vi "field emission sensor_v57.vi"() -> ()   [LabVIEW 2014]
uses:
  Keithley 24XX/Public/Data/Read (Single Point).vi
  Keithley 24XX/Keithley 24XX.lvlib
  <userlib>/Nanonis Prog Interface V5/Nanonis Prog Interface.lvlib
panel:
  out "amplitude":sgl(graph)
  in  "delay  coarse step":u32
  in  "Amplitude (V) (NaN=no change)":sgl=nan
  in  "Frequency (Hz) (NaN=no change)":sgl=nan format="%#_6p"
  in  "retract":dbl=2e-08 format="%#_6p"
  in  "amplitude max":sgl=1e-10 format="%#_6p"
  in  "Signal index (0-79)":i8=49
  out "amplitude":sgl=7.943678e-12 format="%#_6p"
  in  "dz":dbl=1e-09 format="%#_6p"
  in  "ramp delay":u16=10500
  out "ramp":bool
  out "millisecond timer value":u32=183946603
  in  "Clear plots":bool
  out "z":dbl(graph)=1.0959994182086754e-07
  in  "Ramp":bool=TRUE
  in  "steps":sgl=5e-09 format="%#_6p"
  in  "Ramp to":sgl=2.45e-07 format="%#_6p"
  in  "I":sgl=5e-05 format="%#_6p"
  in  "PID":bool
  in  "p":sgl=0.005 format="%#_6p"
  in  "setpoint":sgl=2.5000006e-07 format="%#_6p"
  in  "max Current":sgl=1e-06 format="%#_6p"
  in  "setpoint approach":sgl=3e-08 format="%#_6p"
  in  "auto approach":bool
  in  "Number of steps":u16=1
  in  "withdraw tip":bool
  in  "coarse step":bool
  in  "Direction":enum16{"X +", "X -", "Y +", "Y -", "Z +", "Z -"}(ring)=enum."Z +"
  in  "Machine name (local machine IP)":string="localhost"
  in  "Z position [m]":dbl=1.0959994182086754e-07 step=1.0 format="%_6p"
  out "current [A]":sgl=2.086008e-11 format="%#_6p"
  in  "time divider":dbl=60.0
  out "time elapsed":dbl=58.44645961125692
  in  "milliseconds to wait":u32=100
  in  "VISA resource name":refnum<visa-resource-name>="GPIB0::21::INSTR"
  in  "stop":bool
  in  "current multiplier":sgl=1.0
  out "Current":sgl(graph)=2.086008e-11
  # "STOP the VI during an Nanonis Auto Approach"
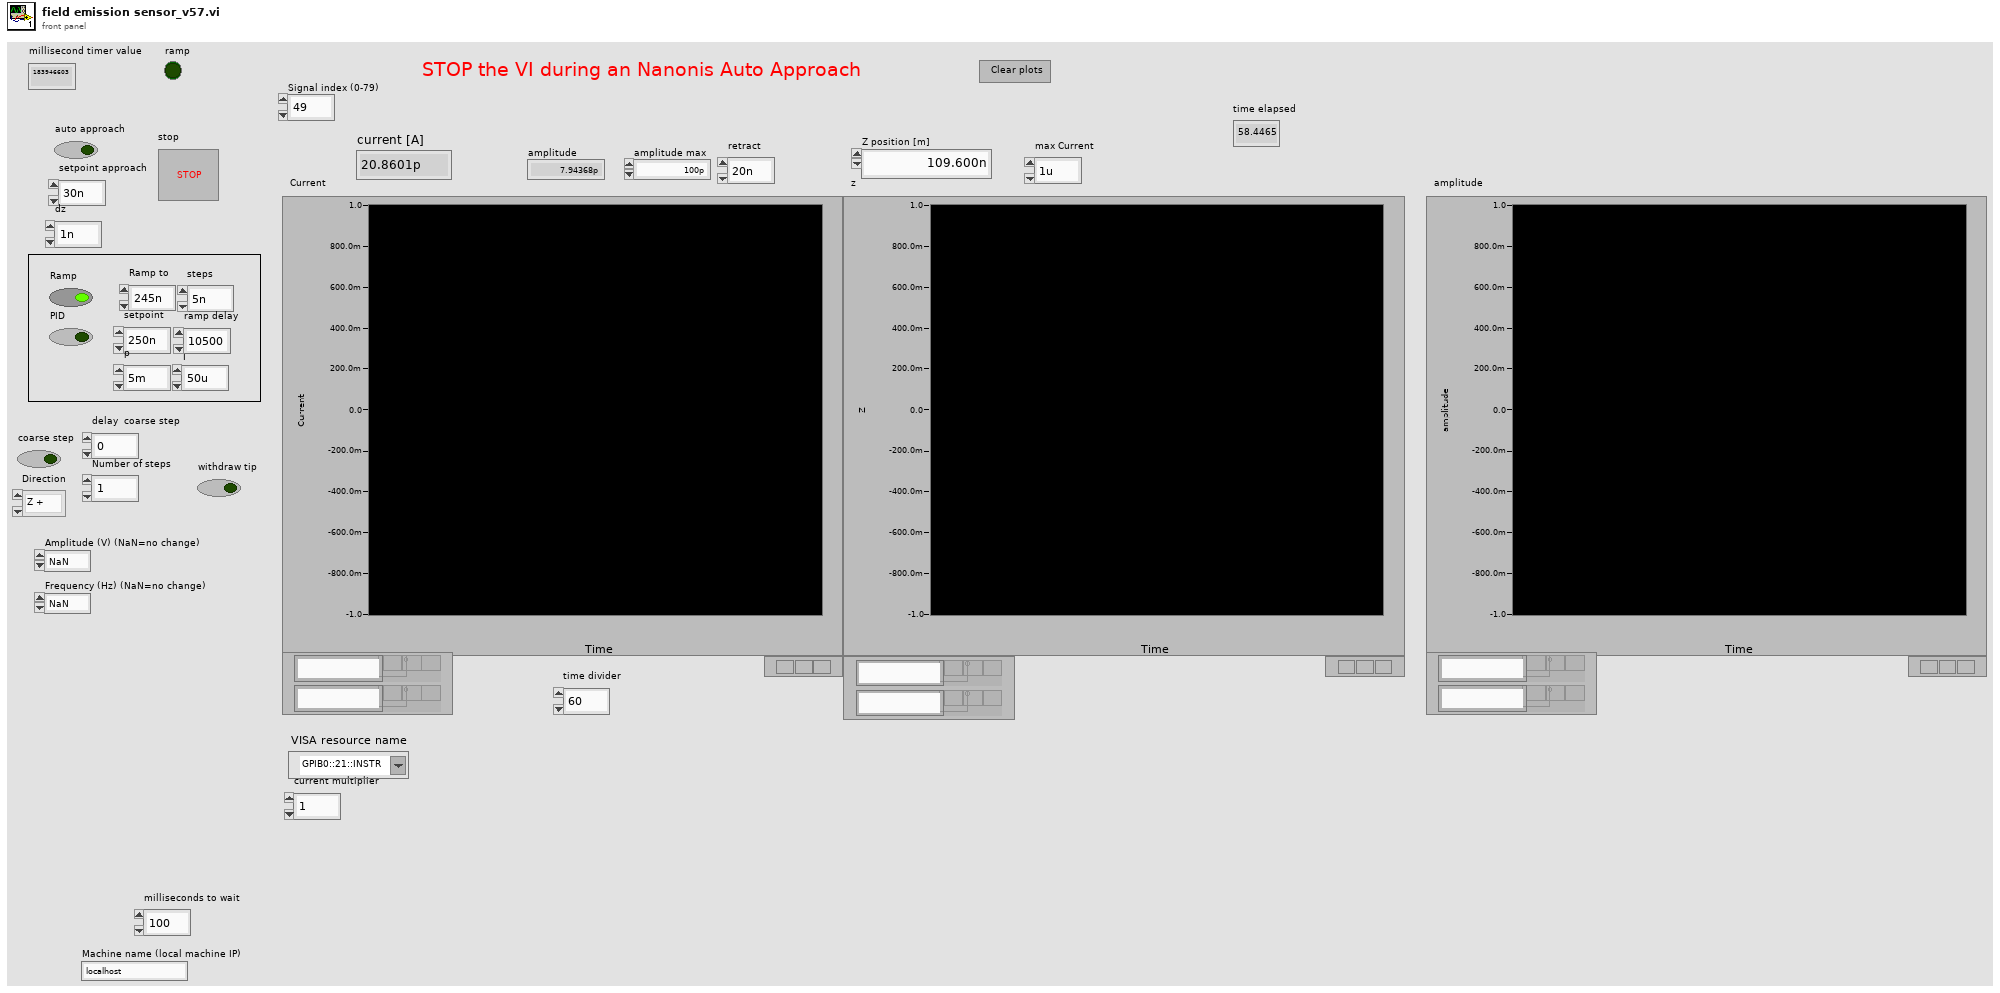
[diagram p1: front panel]
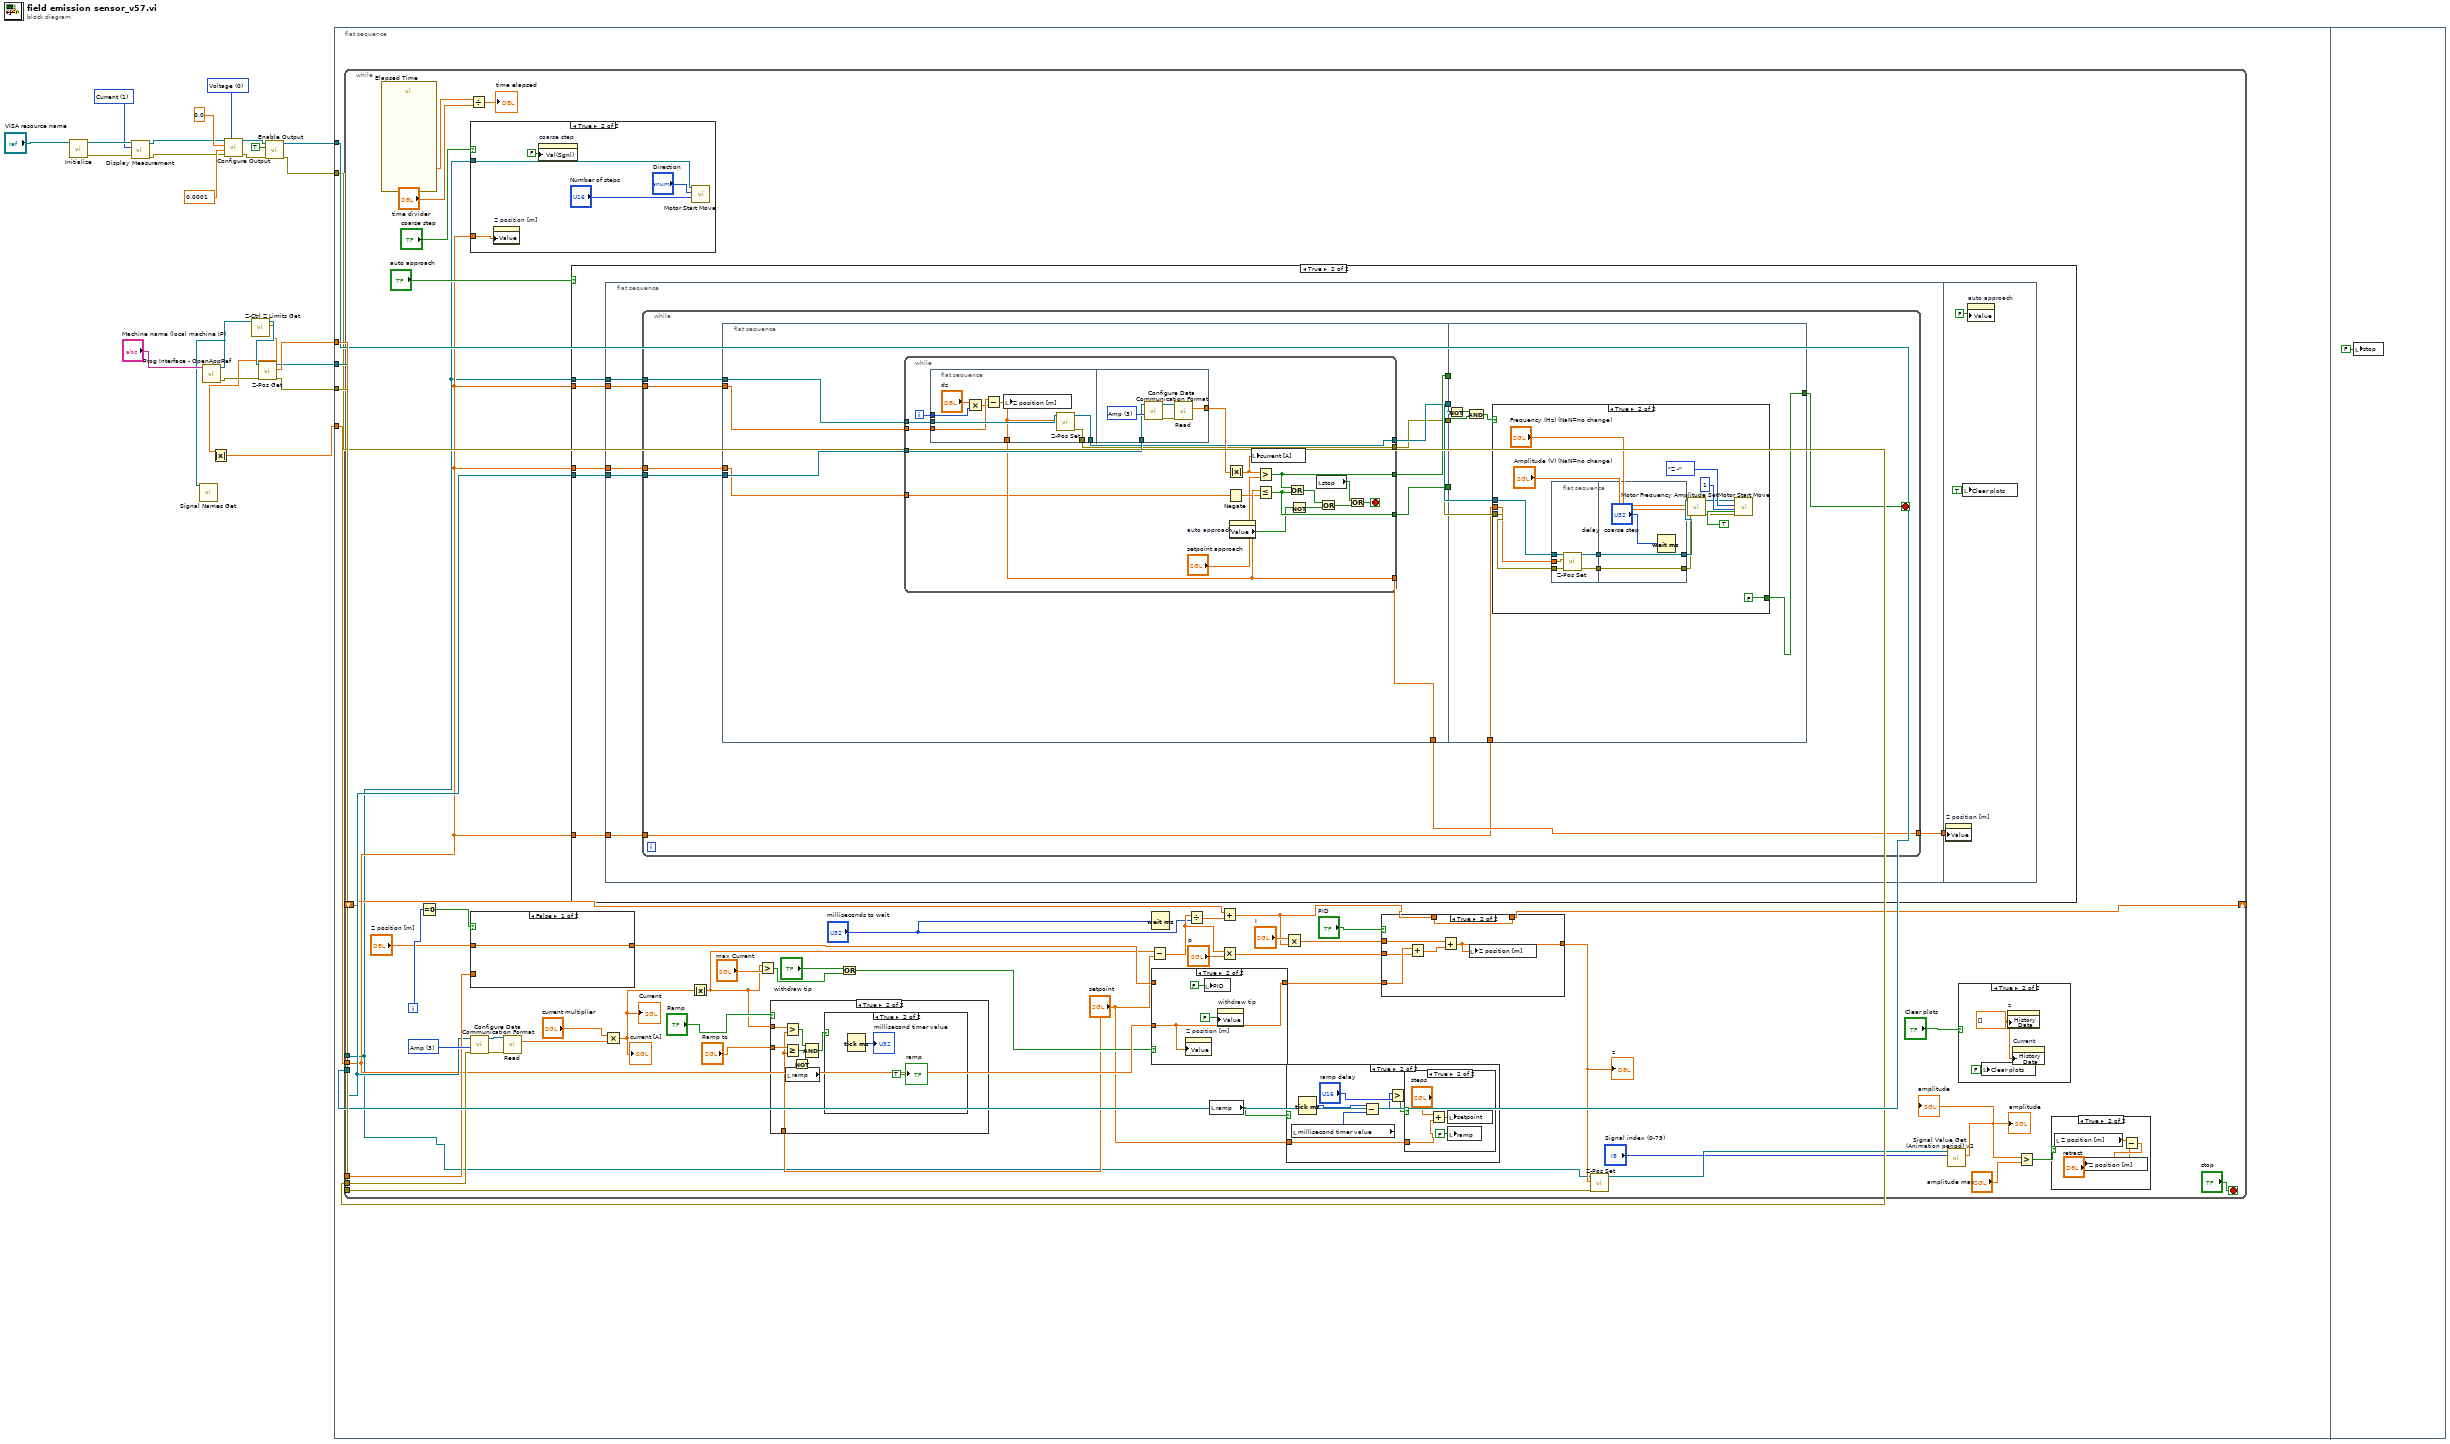
[diagram p0: block diagram]
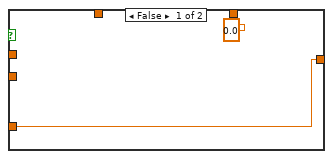
[diagram p8: hidden frame]
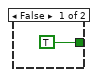
[diagram p10: hidden frame]
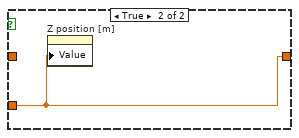
[diagram p13: hidden frame]
diagram:
  w5 = u16 1 items=["Voltage", "Current", "Resistance"] ("Displayed Measurement (0: Voltage)")
  w17 = u16 0 items=["Voltage", "Current"] ("Source Mode  (0: Voltage)")
  n1 = call "Initialize.vi"("VISA resource name"="VISA resource name") -> ("error out"=w7:errorcluster, "VISA resource name out"=w9:refnum<visa-resource-name>)  [unwired: 9 in]
  n2 = call "Display Measurement.vi"("error in (no error)"=w7, "Displayed Measurement (0: Voltage)"=w5, "VISA resource name"=w9) -> ("error out"=w6:errorcluster, "VISA resource name out"=w8:refnum<visa-resource-name>)  [unwired: 7 in]
  n3 = call <userlib>:"Prog Interface - OpenAppRef.vi"("Machine name (local machine IP)"="Machine name (local machine IP)") -> ("Error out"=w22:errorcluster, "Application reference"=w1:refnum<vi>)  [unwired: 5 in]
  n4 = call <userlib>:"Signal Names Get.vi"("Application ref in"=w1) -> ()  [unwired: 6 in, 3 out]
  n5 = call "Configure Output.vi"("Source Mode  (0: Voltage)"=w17, "error in (no error)"=w6, "Compliance  Level (0.1)"=0.0001, "Output Level (0)"=0.0, "VISA resource name"=w8) -> ("error out"=w13:errorcluster, "VISA resource name out"=w14:refnum<visa-resource-name>)  [unwired: 5 in]
  n6 = call <userlib>:"Z-Ctrl Z Limits Get.vi"("Application ref in"=w1) -> ("Z high limit"=w2:sgl, "Application ref out"=w3:refnum<vi>)  [unwired: 7 in, 2 out]
  n7 = Absolute Value(x=w2) -> (abs(x)=w4:sgl)
  n8 = call <userlib>:"Z-Pos Get.vi"("error in (no error)"=w22, "Application ref in"=w3) -> ("error out"=w21:errorcluster, "Z position (m)"=w20:sgl, "Application ref out"=w19:refnum<vi>)  [unwired: 7 in]
  n9 = call "Enable Output.vi"("error in (no error)"=w13, "Enable Output (T: Enable)"=TRUE, "VISA resource name"=w14) -> ("error out"=w10:errorcluster, "VISA resource name out"=w11:refnum<visa-resource-name>)  [unwired: 7 in]
  n10 = flat-sequence {
    tunnel: w21 -> [w29]
    tunnel: w20 -> [w28]
    tunnel: w19 -> [w27]
    tunnel: w11 -> [w26]
    tunnel: w10 -> [w25]
    tunnel: w4 -> [w24]
    frame #0 {
      n11 = while {
        tunnel: w27 -> [w33]
        tunnel: w29 -> [w71]
        tunnel: w28 -> [w70]
        tunnel: w26 -> [w62]
        tunnel: w25 -> [w61]
        tunnel: w24 -> [w59]
        shift-right: [w43] -> _
        shift-left: _ -> [w50]
        i -> [w69]
        stop <- "stop" stop-if-true
        w75 = u16 3 items=["All", "Volt and Amp", "Volt", "Amp"] ("Data Selection (0: All)")
        n12 = call "Elapsed Time"() -> ("Elapsed Time (s)"=w72:dbl)  [unwired: 12 in, 7 out]
        n13 = Equal To 0?(x=w69) -> (x = 0?=w68:bool)
        n14 = Divide(x=w72, y="time divider") -> (x/y=→"time elapsed":dbl)
        n15 = case shown="True" "coarse step" {
          tunnel: w33 -> [_ w221]
          tunnel: w59 -> [_ w217]
          frame False {
          }
          frame True {
            n16 = property on="Z position [m]" class="DigNum (strict)"("Value"=w217) -> ()  [unwired: 2 in, 2 out]
            n17 = property on="coarse step" class="Bool (strict)"("Val(Sgnl)"=FALSE ("Value (Signaling)")) -> ()  [unwired: 2 in, 2 out]
            n18 = call <userlib>:"Motor Start Move.vi"("Number of steps"="Number of steps", "Direction"="Direction", "Application ref in"=w221) -> ()  [unwired: 6 in, 2 out]
          }
        }
        n19 = case shown="False" w68 {
          tunnel: [w222 w223] -> w65
          tunnel: w70 -> [_ w223]
          tunnel: "Z position [m]" -> [w222 _]
          frame False {
          }
          frame True {
            n20 = property on="Z position [m]" class="DigNum (strict)"("Value"=w223) -> ()  [unwired: 2 in, 2 out]
          }
        }
        n21 = call "Configure Data Communication Format.vi"("error in (no error)"=w61, "Data Selection (0: All)"=w75, "VISA resource name"=w62) -> ("error out"=w76:errorcluster, "VISA resource name out"=w77:refnum<visa-resource-name>)  [unwired: 7 in]
        n22 = call-poly "Read.vi"("VISA resource name"=w77, "error in (no error)"=w76) -> ("Current"=w79:sgl)  [unwired: 7 in, 6 out]
        n23 = case shown="True" "auto approach" {
          tunnel: w62 -> [_ w118]
          tunnel: w33 -> [_ w117]
          tunnel: w59 -> [_ w115]
          tunnel: w59 -> [_ w114]
          tunnel: w59 -> [_ w113]
          frame False {
          }
          frame True {
            n24 = flat-sequence {
              tunnel: w118 -> [w124]
              tunnel: w117 -> [w123]
              tunnel: [w122] -> w116
              tunnel: w115 -> [w121]
              tunnel: w114 -> [w120]
              tunnel: w113 -> [w119]
              tunnel: w116 -> [w211]
              frame #0 {
                n25 = while {
                  tunnel: w124 -> [w135]
                  tunnel: w123 -> [w134]
                  tunnel: [w128] -> w122
                  tunnel: w121 -> [w127]
                  tunnel: w120 -> [w126]
                  tunnel: w119 -> [w125]
                  stop <- w129 stop-if-true
                  n26 = flat-sequence {
                    tunnel: w135 -> [w144]
                    tunnel: w134 -> [w143]
                    tunnel: [w142] -> w133
                    tunnel: [w141] -> w132
                    tunnel: [w140] -> w131
                    tunnel: [w139] -> w130
                    tunnel: [w138] -> w128
                    tunnel: w127 -> [w137]
                    tunnel: w125 -> [w136]
                    tunnel: w133 -> [w185]
                    tunnel: w132 -> [w183]
                    tunnel: w131 -> [w181]
                    tunnel: w130 -> [w180]
                    tunnel: [w179] -> w129
                    tunnel: w126 -> [w178]
                    frame #0 {
                      n27 = while {
                        tunnel: w144 -> [w163]
                        tunnel: w143 -> [w161]
                        tunnel: [w160] -> w142
                        tunnel: [w159] -> w141
                        tunnel: [w158] -> w140
                        tunnel: [w157] -> w139
                        tunnel: [w156] -> w138
                        tunnel: w137 -> [w155]
                        tunnel: w136 -> [w153]
                        i -> [w164]
                        stop <- w148 stop-if-true
                        n28 = flat-sequence {
                          tunnel: w164 -> [w172]
                          tunnel: w161 -> [w171]
                          tunnel: [w166] -> w156
                          tunnel: [w170] -> w158
                          tunnel: [w169] -> w157
                          tunnel: w155 -> [w168]
                          tunnel: w163 -> [w174]
                          tunnel: [w173] -> w162
                          frame #0 {
                            n29 = Multiply(x="dz", y=w172) -> (x*y=w167:dbl)
                            n30 = Subtract(x=w168, y=w167) -> (x-y=w166:dbl)
                            n31 = local write "Z position [m]"(w166) -> ()
                            n32 = call <userlib>:"Z-Pos Set.vi"("Z position (m)"=w166, "Application ref in"=w171) -> ("error out"=w169:errorcluster, "Application ref out"=w170:refnum<vi>)  [unwired: 8 in]
                          }
                          frame #1 {
                            w175 = u16 3 items=["All", "Volt and Amp", "Volt", "Amp"] ("Data Selection (0: All)")
                            n33 = call "Configure Data Communication Format.vi"("Data Selection (0: All)"=w175, "VISA resource name"=w174) -> ("error out"=w176:errorcluster, "VISA resource name out"=w177:refnum<visa-resource-name>)  [unwired: 8 in]
                            n34 = call-poly "Read.vi"("VISA resource name"=w177, "error in (no error)"=w176) -> ("Current"=w173:sgl)  [unwired: 7 in, 6 out]
                          }
                        }
                        n35 = Negate(x=w153) -> (-x=w154:sgl)
                        n36 = Absolute Value(x=w162) -> (abs(x)=w145:sgl)
                        n37 = property on="auto approach" class="Bool (strict)"() -> ("Value"=w151:bool)  [unwired: 2 in, 2 out]
                        n38 = local write "current [A]"(w145) -> ()
                        n39 = Greater?(x=w145, y="setpoint approach") -> (0:w160:bool)
                        n40 = Less Or Equal?(x=w156, y=w154) -> (x <= y?=w159:bool)
                        n41 = Or(x=w160, y=w159) -> (x .or. y?=w152:bool)
                        n42 = Not(x=w151) -> (.not. x?=w150:bool)
                        n43 = local read "stop"() -> (w147:bool)
                        n44 = Or(x=w152, y=w150) -> (x .or. y?=w149:bool)
                        n45 = Or(x=w147, y=w149) -> (x .or. y?=w148:bool)
                      }
                    }
                    frame #1 {
                      n46 = Not(x=w185) -> (.not. x?=w184:bool)
                      n47 = And(x=w184, y=w183) -> (x .and. y?=w182:bool)
                      n48 = case shown="True" w182 {
                        tunnel: w181 -> [_ w201]
                        tunnel: w180 -> [_ w200]
                        tunnel: [TRUE FALSE] -> w179
                        tunnel: w178 -> [_ w196]
                        frame False {
                        }
                        frame True {
                          n49 = flat-sequence {
                            tunnel: w201 -> [w206]
                            tunnel: w200 -> [w205]
                            tunnel: w196 -> [w204]
                            tunnel: [w203] -> w188
                            tunnel: [w202] -> w187
                            tunnel: [w208] -> w192
                            tunnel: [w209] -> w193
                            tunnel: w188 -> [w209]
                            tunnel: w187 -> [w208]
                            frame #0 {
                              n50 = call <userlib>:"Z-Pos Set.vi"("error in (no error)"=w205, "Z position (m)"=w204, "Application ref in"=w206) -> ("error out"=w202:errorcluster, "Application ref out"=w203:refnum<vi>)  [unwired: 7 in]
                            }
                            frame #1 {
                              n51 = Wait (ms)(milliseconds to wait="delay  coarse step") -> ()  [unwired: 1 out]
                            }
                          }
                          n52 = call <userlib>:"Motor Frequency Amplitude Set.vi"("Error in (no error)"=w192, "Amplitude (V) (NaN=no change)"="Amplitude (V) (NaN=no change)", "Frequency (Hz) (NaN=no change)"="Frequency (Hz) (NaN=no change)", "Application ref in"=w193) -> ("Error out"=w191:errorcluster, "Application ref out"=w194:refnum<vi>)  [unwired: 6 in]
                          n53 = call <userlib>:"Motor Start Move.vi"("Wait until finished? (F)"=TRUE, "Error in (no error)"=w191, "Number of steps"=u16 1, "Direction"=enum16{"X +", "X -", "Y +", "Y -", "Z +", "Z -"}."Z -", "Application ref in"=w194) -> ()  [unwired: 4 in, 2 out]
                        }
                      }
                    }
                  }
                }
              }
              frame #1 {
                n54 = property on="Z position [m]" class="DigNum (strict)"("Value"=w211) -> ()  [unwired: 2 in, 2 out]
                n55 = local write "Clear plots"(TRUE ("Clear plots")) -> ()
                n56 = property on="auto approach" class="Bool (strict)"("Value"=FALSE ("auto approach")) -> ()  [unwired: 2 in, 2 out]
              }
            }
          }
        }
        n57 = Multiply(x="current multiplier", y=w79) -> (x*y=w58:sgl)
        "Current" <- w58
        "current [A]" <- w58
        n58 = Absolute Value(x=w58) -> (abs(x)=w41:sgl)
        n59 = Greater?(x=w41, y="max Current") -> (0:w55:bool)
        n60 = case shown="True" "Ramp" {
          tunnel: w41 -> [_ w102]
          tunnel: "setpoint" -> [_ w99]
          tunnel: "Ramp to" -> [_ w100]
          frame False {
          }
          frame True {
            n61 = Greater?(x=w102, y=w99) -> (0:w101:bool)
            n62 = Greater Or Equal?(x=w100, y=w99) -> (x >= y?=w97:bool)
            n63 = local read "ramp"() -> (w96:bool)
            n64 = Not(x=w96) -> (.not. x?=w95:bool)
            n65 = Compound Arithmetic op=AND(w101, w97, w95) -> (w98:bool)
            n66 = case shown="True" w98 {
              frame False {
              }
              frame True {
                n67 = Tick Count (ms)() -> (millisecond timer value=→"millisecond timer value":u32)
                "ramp" <- TRUE ("ramp")
              }
            }
          }
        }
        n68 = Or(x="withdraw tip", y=w55) -> (x .or. y?=w56:bool)
        n69 = Subtract(x=w41, y="setpoint") -> (x-y=w46:sgl)
        n70 = Wait (ms)(milliseconds to wait="milliseconds to wait") -> ()  [unwired: 1 out]
        n71 = case shown="True" w56 {
          tunnel: [w213 w215] -> w52
          tunnel: w65 -> [w213 _]
          tunnel: w59 -> [_ w215]
          frame False {
          }
          frame True {
            n72 = property on="Z position [m]" class="DigNum (strict)"("Value"=w215) -> ()  [unwired: 2 in, 2 out]
            n73 = local write "PID"(FALSE ("PID")) -> ()
            n74 = property on="withdraw tip" class="Bool (strict)"("Value"=FALSE ("withdraw tip")) -> ()  [unwired: 2 in, 2 out]
          }
        }
        n75 = Divide(x=w46, y="milliseconds to wait") -> (x/y=w47:sgl)
        n76 = local read "ramp"() -> (w36:bool)
        n77 = Add(x=w50, y=w47) -> (x+y=w44:sgl)
        n78 = Multiply(x=w46, y="p") -> (x*y=w51:sgl)
        n79 = Multiply(x="I", y=w44) -> (x*y=w48:sgl)
        n80 = case shown="True" w36 {
          tunnel: "setpoint" -> [_ w83]
          frame False {
          }
          frame True {
            n81 = local read "millisecond timer value"() -> (w87:u32)
            n82 = Tick Count (ms)() -> (millisecond timer value=w88:u32)
            n83 = Subtract(x=w88, y=w87) -> (x-y=w85:u32)
            n84 = Greater?(x=w85, y="ramp delay") -> (0:w84:bool)
            n85 = case shown="True" w84 {
              tunnel: w83 -> [_ w90]
              frame False {
              }
              frame True {
                n86 = Add(x="steps", y=w90) -> (x+y=w92:sgl)
                n87 = local write "setpoint"(w92) -> ()
                n88 = local write "ramp"(FALSE ("ramp")) -> ()
              }
            }
          }
        }
        n89 = case shown="True" "PID" {
          tunnel: w52 -> [w106 w112]
          tunnel: [w106 w108] -> w39
          tunnel: w51 -> [_ w111]
          tunnel: w48 -> [_ w109]
          tunnel: w44 -> [_ w107]
          tunnel: [sgl 0.0 w107] -> w43
          frame False {
          }
          frame True {
            n90 = Add(x=w112, y=w111) -> (x+y=w110:dbl)
            n91 = Add(x=w109, y=w110) -> (x+y=w108:dbl)
            n92 = local write "Z position [m]"(w108) -> ()
          }
        }
        "z" <- w39
        n93 = call <userlib>:"Z-Pos Set.vi"("error in (no error)"=w71, "Z position (m)"=w39, "Application ref in"=w33) -> ("Application ref out"=w35:refnum<vi>)  [unwired: 7 in, 1 out]
        n94 = call <userlib>:"Signal Value Get (Animation period) v2.vi"("Signal index (0-79)"="Signal index (0-79)", "Application ref in"=w35) -> ("Signal value"=w30:sgl)  [unwired: 6 in, 2 out]
        "amplitude" <- w30
        "amplitude" <- w30
        n95 = case shown="True" "Clear plots" {
          frame False {
          }
          frame True {
            w94 = dbl[] [] ("History Data")
            n96 = local write "Clear plots"(FALSE ("Clear plots")) -> ()
            n97 = property on="z" class="WFChart (strict)"("History Data"=w94) -> ()  [unwired: 2 in, 2 out]
            n98 = property on="Current" class="WFChart (strict)"("History Data"=w94) -> ()  [unwired: 2 in, 2 out]
          }
        }
        n99 = Greater?(x=w30, y="amplitude max") -> (0:w31:bool)
        n100 = case shown="True" w31 {
          frame False {
          }
          frame True {
            n101 = local read "Z position [m]"() -> (w82:dbl)
            n102 = Subtract(x=w82, y="retract") -> (x-y=w81:dbl)
            n103 = local write "Z position [m]"(w81) -> ()
          }
        }
      }
    }
    frame #1 {
      n104 = local write "stop"(FALSE ("stop")) -> ()
    }
  }
